vi "Base_eleve.vi"() -> ()   [LabVIEW 2018]
uses:
  <vilib>/Instr/_visa.llb/VISA Configure Serial Port (Instr).vi
panel:
  out "Array":dbl[](array[numeric])
  out "Numeric":dbl
  out "Waveform Chart 3":dbl(graph)
  out "Waveform Chart 2":dbl(graph)
  out "Waveform Chart":dbl(graph)
  out "Humidité Moyenne":string
  out "Humidité MIN":string
  out "Humidité MAX":string
  out "Humidité":string
  out "Préssion Moyenne":string
  out "Préssion MIN":string
  out "Pression MAX":string
  out "Presion":string
  out "Température moyenne":string
  out "Température MIN":string
  out "Température MAX":string
  out "Température":string
  in  "stop":bool
  in  "Nom de ressource VISA":refnum<visa-resource-name>
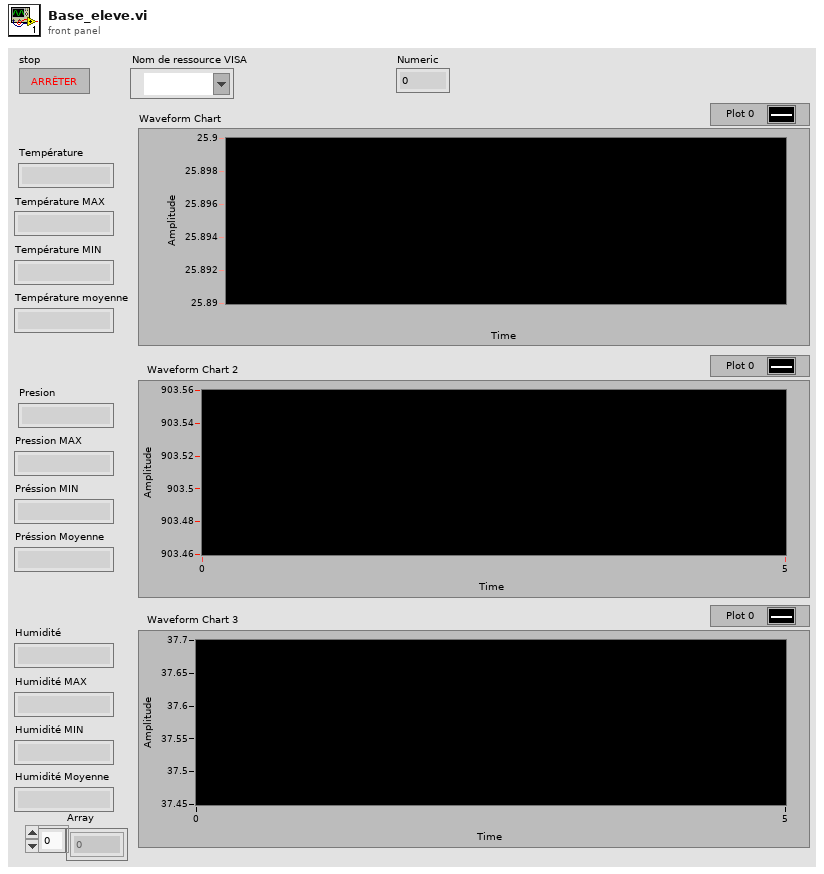
[diagram p1: front panel]
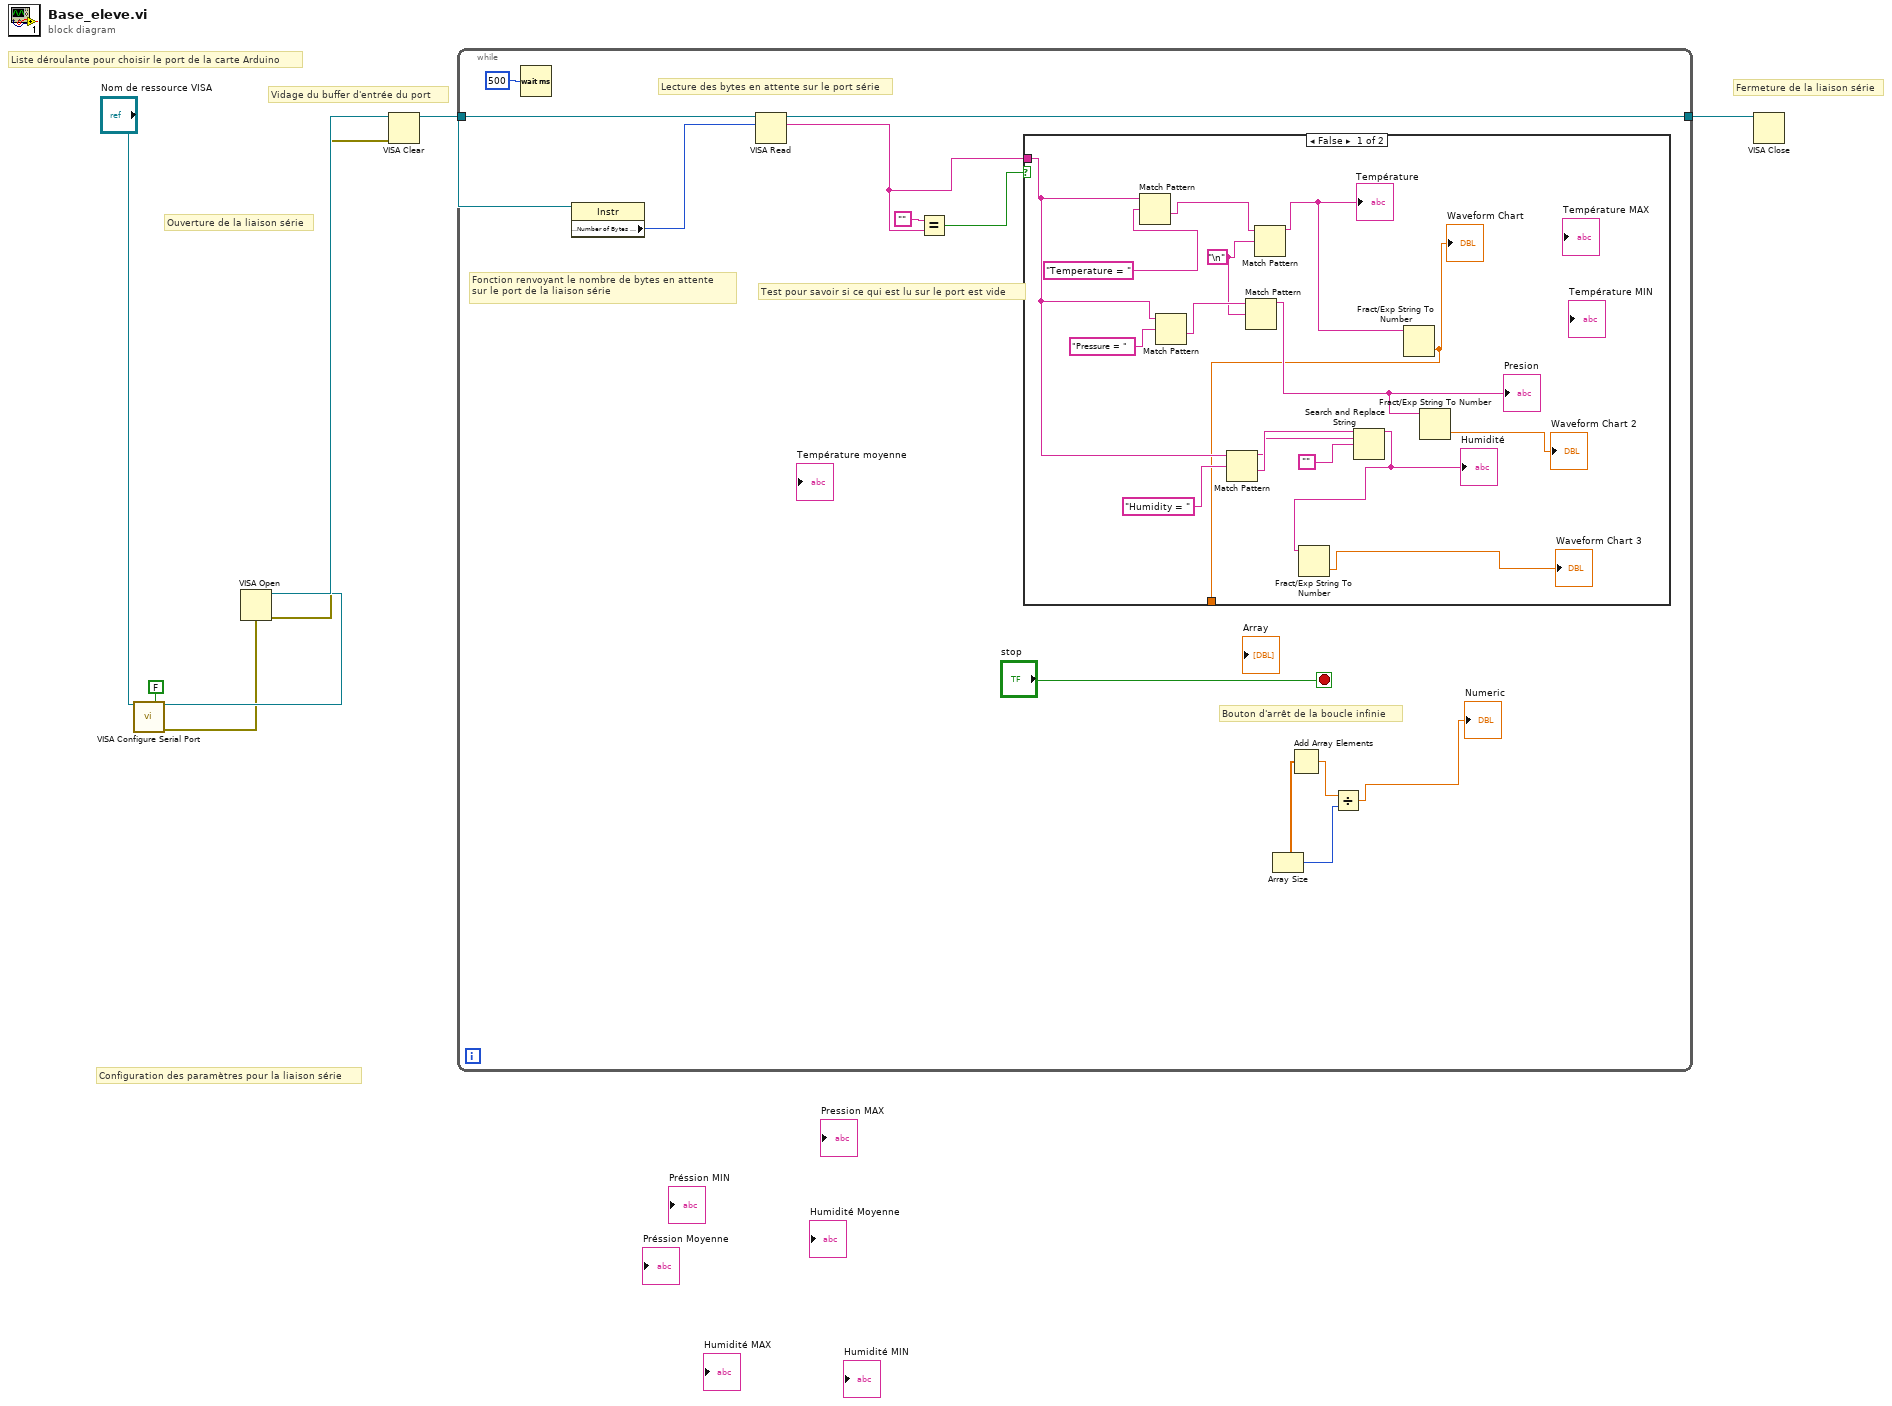
[diagram p0: block diagram]
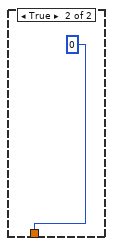
[diagram p2: hidden frame]
diagram:
  # "Vidage du buffer d'entrée du port"
  # "Ouverture de la liaison série"
  # "Configuration des paramètres pour la liaison série"
  # "Liste déroulante pour choisir le port de la carte Arduino"
  # "Fermeture de la liaison série"
  n1 = call-poly "VISA Configure Serial Port"("VISA resource name"="Nom de ressource VISA", "Enable Termination\nChar (T)"=FALSE ("Enable Termination\nChar (T)")) -> ("VISA resource name out"=w5:refnum<visa-resource-name>, "error out"=w3:errorcluster)  [unwired: 12 in]
  n2 = VISA Open(error in (no error)=w3, VISA resource name=w5) -> (VISA resource name=w7:refnum<visa-resource-name>, error out=w2:errorcluster)  [unwired: 3 in]
  n3 = VISA Clear(VISA resource name=w7, error in (no error)=w2) -> (VISA resource name out=w6:refnum<visa-resource-name>)  [unwired: 1 out]
  n4 = while {
    tunnel: w6 -> [w19]
    tunnel: [w17] -> w1
    stop <- "stop" stop-if-true
    # "Lecture des bytes en attente sur le port série"
    # "Fonction renvoyant le nombre de bytes en attente\nsur le port de la liaison série"
    # "Test pour savoir si ce qui est lu sur le port est vide"
    # "Bouton d'arrêt de la boucle infinie"
    n5 = Wait (ms)(milliseconds to wait=u32 500 ("attente (ms)")) -> ()  [unwired: 1 out]
    n6 = property class="Instr"(reference=w19) -> ("Serial Settings:Number of Bytes at Serial Port"=w18:u32)  [unwired: 1 in, 2 out]
    n7 = VISA Read(VISA resource name=w19, byte count=w18) -> (VISA resource name out=w17:refnum<visa-resource-name>, read buffer=w13:string)  [unwired: 1 in, 2 out]
    n8 = Equal?(x="", y=w13) -> (x = y?=w14:bool)
    n9 = case shown="False" w14 {
      tunnel: w13 -> [w30 _]
      tunnel: [w21 0] -> _
      frame False {
        w27 = "\n"
        n10 = Match Pattern(string=w30, regular expression="Temperature = ") -> (after substring=w31:string)  [unwired: 1 in, 3 out]
        n11 = Match Pattern(string=w30, regular expression="Pressure = ") -> (after substring=w28:string)  [unwired: 1 in, 3 out]
        n12 = Match Pattern(string=w30, regular expression="Humidity = ") -> (before substring=w35:string, after substring=w36:string)  [unwired: 1 in, 2 out]
        n13 = Match Pattern(string=w28, regular expression=w27) -> (before substring=w25:string)  [unwired: 1 in, 3 out]
        "Presion" <- w25
        n14 = Match Pattern(string=w31, regular expression=w27) -> (before substring=w24:string)  [unwired: 1 in, 3 out]
        "Température" <- w24
        n15 = Search and Replace String(input string=w36, search string=w35, replace string="") -> (result string=w26:string)  [unwired: 5 in, 3 out]
        "Humidité" <- w26
        n16 = Fract/Exp String To Number(string=w26) -> (number=→"Waveform Chart 3":dbl)  [unwired: 3 in, 1 out]
        n17 = Fract/Exp String To Number(string=w24) -> (number=w21:dbl)  [unwired: 3 in, 1 out]
        "Waveform Chart" <- w21
        n18 = Fract/Exp String To Number(string=w25) -> (number=→"Waveform Chart 2":dbl)  [unwired: 3 in, 1 out]
      }
      frame True {
      }
    }
    n19 = Add Array Elements() -> (numeric array=w9:dbl[], sum=w12:dbl)
    n20 = Array Size(array=w9) -> (size(s)=w11:i32)
    n21 = Divide(x=w12, y=w11) -> (x/y=→"Numeric":dbl)
  }
  n22 = VISA Close(VISA resource name=w1) -> ()  [unwired: 1 in, 1 out]
